vi "Image position, rotation and scale.vi"(0 "Watermark cluster IN":T1={"Show? (F)"=TRUE, "Type"=enum."Image", "Opacity (%)"=10.0, "Rotate(°)"=0.0, "Position"={"Position"=enum."Center (text section)", "X"=0.0, "Y"=0.0}, "Image path"=path "", "Scaled(%)"=100.0, "Image refnum"=refnum, "Text"="CONFIDENTIAL", "Font"={"Name"="", "Size"=-1.0, "Color"=0}, "Font refnum"=refnum, "Alignment"=enum."Center", "Automatic"=FALSE}, 11 "error in (no error)":errorcluster) -> (4 "Watermark cluster OUT":T1={"Show? (F)"=TRUE, "Type"=enum."Image", "Opacity (%)"=10.0, "Rotate(°)"=0.0, "Position"={"Position"=enum."Center (text section)", "X"=0.0, "Y"=0.0}, "Image path"=path "", "Scaled(%)"=100.0, "Image refnum"=refnum, "Text"="CONFIDENTIAL", "Font"={"Name"="", "Size"=-1.0, "Color"=0}, "Font refnum"=refnum, "Alignment"=enum."Center", "Automatic"=FALSE}, 15 "error out":errorcluster)   [LabVIEW 2019, in "Exaprom PDF.lvlib"]
doc: "Version 1.0\nDeveloped by Jean-Marc Simard\nCopyright © 2010, Exaprom Inc.\nAll rights reserved.\nLicense: BSD\n\nWith iTextSharp 4.1.6 (http://itextsharp.sourceforge.net)\nunder Mozilla Public License Version 1.1\n(http://www.mozilla.org/MPL/MPL-1.1.html)"
uses:
  Controls/Header, Footer and Watermark Controls/Watermark cluster2.ctl
  Controls/Header, Footer and Watermark Controls/Watermark Position.ctl
  C:/work/niobrara_lv/labview pdf writer fixing/DLL/itextsharp.dll
  DLL/itextsharp.dll
  Controls/Font Controls/Font size.ctl
  Controls/Font Controls/Font color.ctl
  Controls/Header, Footer and Watermark Controls/Header footer horiz alignment.ctl
  Exaprom PDF.lvlib
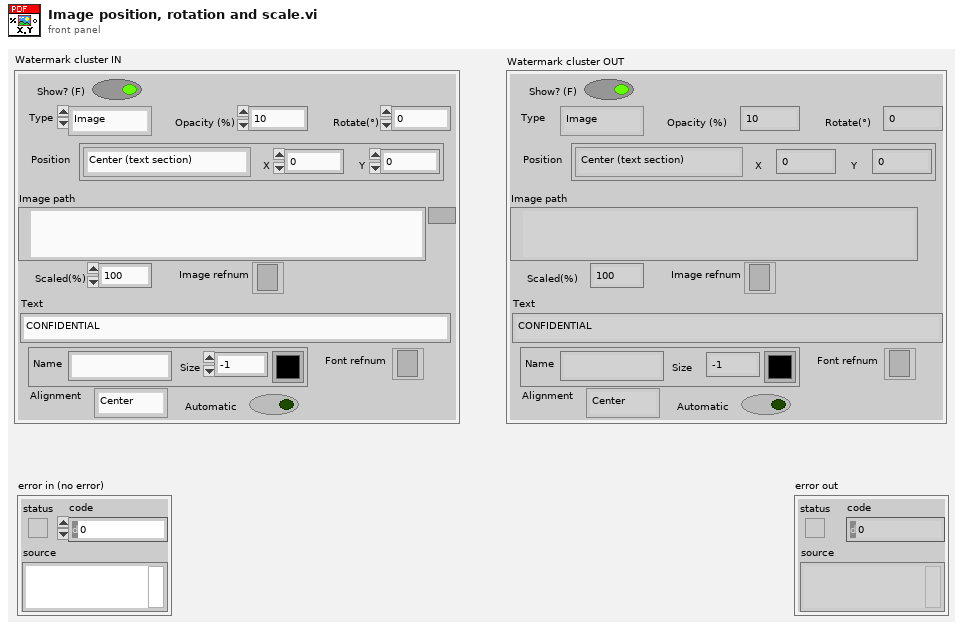
[diagram p1: front panel]
types:
  T1 = typedef "Exaprom PDF.lvlib/Watermark cluster2.ctl" = cluster{"Show? (F)":bool, "Type":enum16{"Image", "Text"}, "Opacity (%)":sgl, "Rotate(°)":sgl, "Position":cluster{"Position":T2, "X":sgl, "Y":sgl}, "Image path":path, "Scaled(%)":sgl, "Image refnum":refnum<k24>, "Text":string, "Font":cluster{"Name":string, "Size":T3, "Color":T4}, "Font refnum":refnum<k24>, "Alignment":T5, "Automatic":bool}
  T2 = typedef "Exaprom PDF.lvlib/Watermark Position.ctl" = enum16{"Absolute", "Center (page)", "Center (text section)"}
  T3 = typedef "Exaprom PDF.lvlib/Font size.ctl" = sgl
  T4 = typedef "Exaprom PDF.lvlib/Font color.ctl" = u32
  T5 = typedef "Exaprom PDF.lvlib/Header footer horiz alignment.ctl" = enum16{"Left", "Center", "Right"}
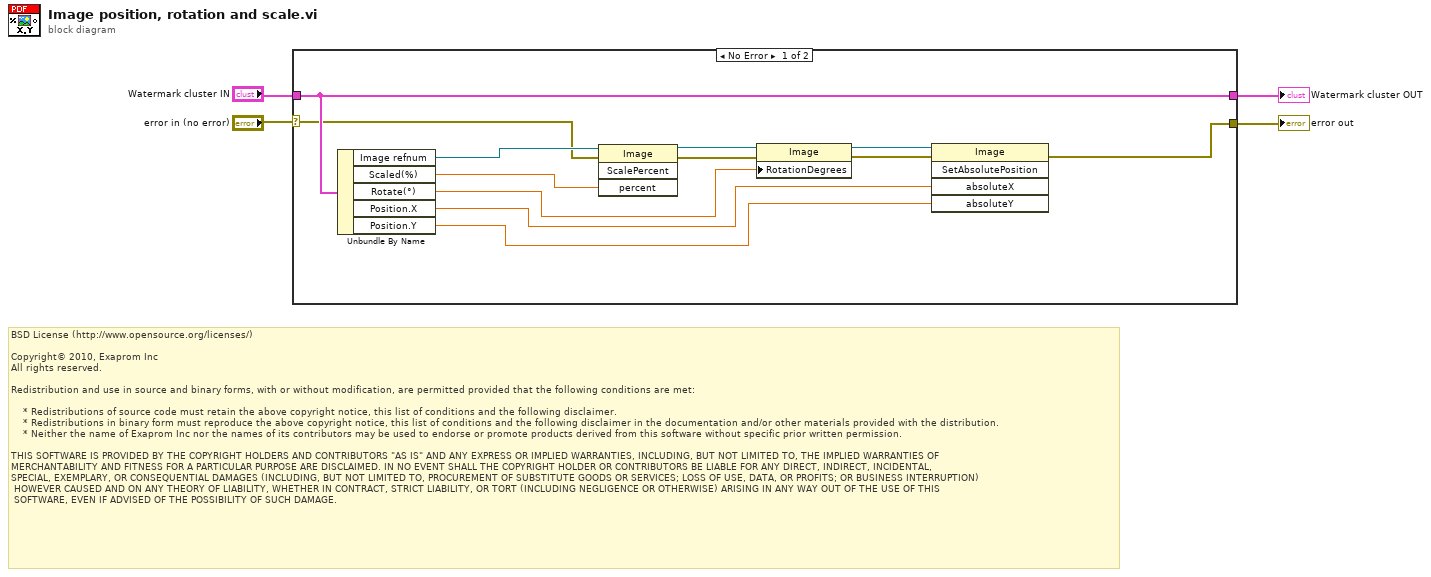
[diagram p0: block diagram]
diagram:
  # "BSD License (http://www.opensource.org/licenses/)\n\nCopyright© 2010, Exaprom Inc\nAll rights reserved.\n\nRedistribution and use in source and binary forms, with or without modification, are permitted provided that the following conditions are met:\n\n    * Redistributions of source code must retain the above copyright notice, this list of conditions and the following disclaimer.\n    * Redistributions in binary form must reproduce the above copyright notice, this list of conditions and the following disclaimer in the documentation and/or other materials provided with the distribution.\n    * Neither the name of Exaprom Inc nor the names of its contributors may be used to endorse or promote products derived from this software without specific prior written permission.\n\nTHIS SOFTWARE IS PROVIDED BY THE COPYRIGHT HOLDERS AND CONTRIBUTORS \"AS IS\" AND ANY EXPRESS OR IMPLIED WARRANTIES, INCLUDING, BUT NOT LIMITED TO, THE IMPLIED WARRANTIES OF \nMERCHANTABILITY AND FITNESS FOR A PARTICULAR PURPOSE ARE DISCLAIMED. IN NO EVENT SHALL THE COPYRIGHT HOLDER OR CONTRIBUTORS BE LIABLE FOR ANY DIRECT, INDIRECT, INCIDENTAL,\nSPECIAL, EXEMPLARY, OR CONSEQUENTIAL DAMAGES (INCLUDING, BUT NOT LIMITED TO, PROCUREMENT OF SUBSTITUTE GOODS OR SERVICES; LOSS OF USE, DATA, OR PROFITS; OR BUSINESS INTERRUPTION)\n HOWEVER CAUSED AND ON ANY THEORY OF LIABILITY, WHETHER IN CONTRACT, STRICT LIABILITY, OR TORT (INCLUDING NEGLIGENCE OR OTHERWISE) ARISING IN ANY WAY OUT OF THE USE OF THIS\n SOFTWARE, EVEN IF ADVISED OF THE POSSIBILITY OF SUCH DAMAGE."
  n1 = case shown="No Error" "error in (no error)" {
    selector: "error in (no error)" -> [w12 w18]
    tunnel: [w11 w18] -> w1
    tunnel: "Watermark cluster IN" -> [w13 w17]
    tunnel: [w13 w17] -> w3
    frame No Error {
      n2 = Unbundle By Name(w13) -> ("Image refnum"=w16:refnum<k24>, "Scaled(%)"=w15:sgl, "Rotate(°)"=w5:sgl, "Position.X"=w6:sgl, "Position.Y"=w14:sgl)
      n3 = invoke class="Image" method="ScalePercent"(reference=w16, error in=w12, "percent"=w15) -> (reference out=w8:refnum<k24>, error out=w9:errorcluster)  [unwired: 1 in, 2 out]
      n4 = property class="Image"(reference=w8, error in=w9, "RotationDegrees"=w5) -> (reference out=w7:refnum<k24>, error out=w10:errorcluster)
      n5 = invoke class="Image" method="SetAbsolutePosition"(reference=w7, error in=w10, "absoluteX"=w6, "absoluteY"=w14) -> (error out=w11:errorcluster)  [unwired: 1 in, 4 out]
    }
    frame Error {
    }
  }
  "error out" <- w1
  "Watermark cluster OUT" <- w3
